vi "SignIn&Out QR Code.vi"(8 "error in (no error)":errorcluster, 11 "Para":T1={"url"="http://data.watersystem.com.cn:50040", "AccessToken"="equip&GbbVkGRBUSaIfhTSjiolTAP8QMM", "mn"="admin", "isSignIn"=FALSE}) -> (0 "error out":errorcluster, 3 "response":T2)   [LabVIEW 2016, in "opSignIn.lvlib"]
uses:
  opSignIn.lvlib
  <vilib>/httpClient/LabVIEWHTTPClient.lvlib
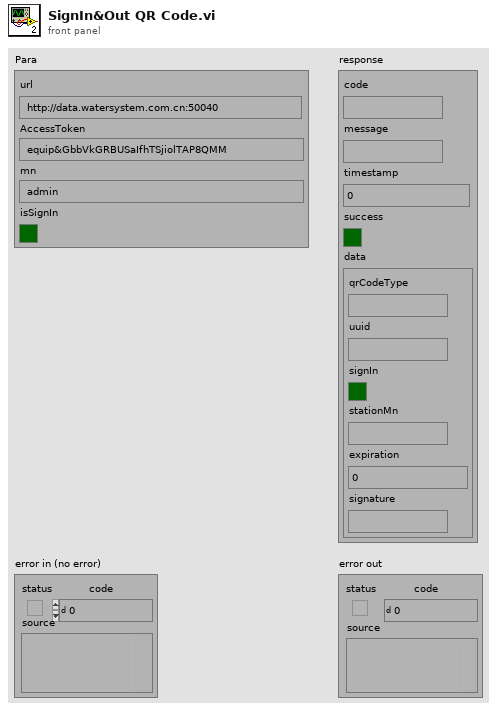
[diagram p1: front panel]
types:
  T1 = cluster{"url":string, "AccessToken":string, "mn":string, "isSignIn":bool}
  T2 = cluster{"code":string, "message":string, "timestamp":u64, "success":bool, "data":cluster{"qrCodeType":string, "uuid":string, "signIn":bool, "stationMn":string, "expiration":u64, "signature":string}}
  T3 = cluster{"code":string, "message":string, "success":bool}
  T4 = typedef "LabVIEWHTTPClient.lvlib/ClientHandle.ctl" = refnum<k1>
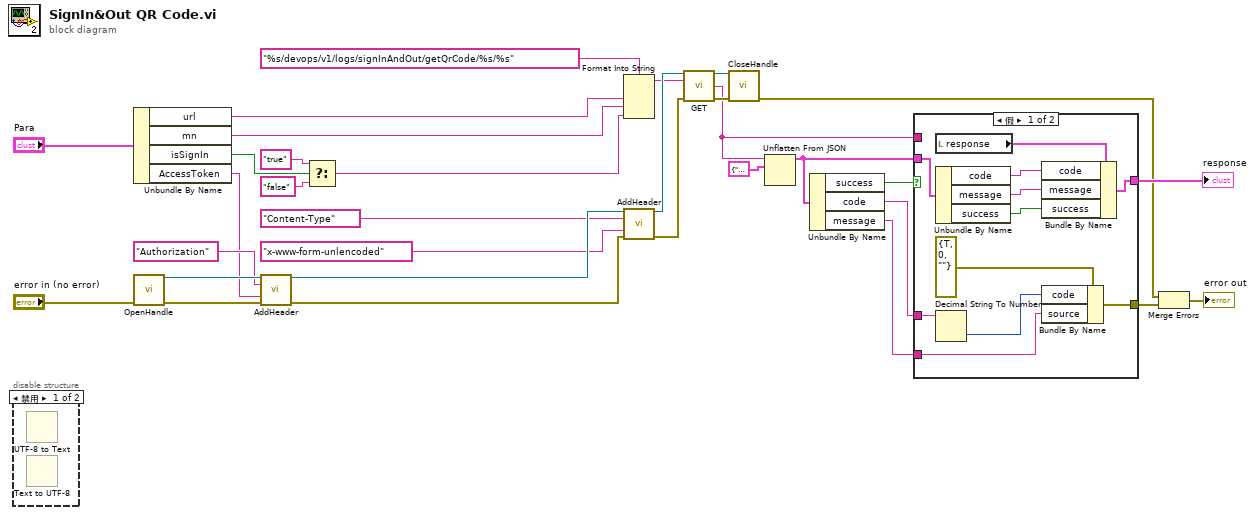
[diagram p0: block diagram]
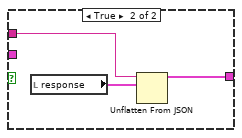
[diagram p2: hidden frame]
diagram:
  n1 = disable-structure shown="禁用" {
    frame Disabled {
      n2 = UTF-8 to Text() -> ()  [unwired: 3 in, 2 out]
      n3 = Text to UTF-8() -> ()  [unwired: 3 in, 2 out]
    }
    frame Enabled {
    }
  }
  n4 = Unbundle By Name("Para") -> ("url"=w1:string, "mn"=w14:string, "isSignIn"=w13:bool, "AccessToken"=w12:string)
  n5 = call <vilib>:"OpenHandle.vi"("error in (no error)"="error in (no error)") -> ("client handle out"=w32:T4, "error out"=w31:errorcluster)  [unwired: 13 in]
  n6 = call <vilib>:"AddHeader.vi"("client handle"=w32, "header"="Authorization", "value"=w12, "error in (no error)"=w31) -> ("client handle out"=w28:T4, "error out"=w27:errorcluster)  [unwired: 10 in]
  n7 = Select(t="true", s=w13, f="false") -> (s? t:f=w16:string)
  n8 = Format Into String(format string="%s/devops/v1/logs/signInAndOut/getQrCode/%s/%s" ("url"), w1, w14, w16) -> (resulting string=w19:string)  [unwired: 2 in, 1 out]
  n9 = call <vilib>:"AddHeader.vi"("client handle"=w28, "header"="Content-Type", "value"="x-www-form-unlencoded", "error in (no error)"=w27) -> ("client handle out"=w24:T4, "error out"=w23:errorcluster)  [unwired: 10 in]
  n10 = call <vilib>:"GET.vi"("client handle"=w24, "url"=w19, "error in (no error)"=w23) -> ("client handle out"=w22:T4, "body"=w8:string, "error out"=w21:errorcluster)  [unwired: 9 in, 1 out]
  n11 = call <vilib>:"CloseHandle.vi"("client handle"=w22, "error in (no error)"=w21) -> ("error out"=w4:errorcluster)  [unwired: 13 in]
  n12 = Unflatten From JSON(JSON string=w8, type and defaults=T3 {"code"="", "message"="", "success"=FALSE} ("response 2")) -> (value=w7:T3)  [unwired: 5 in, 1 out]
  n13 = Unbundle By Name(w7) -> ("success"=w10:bool, "code"=w6:string, "message"=w5:string)
  n14 = case shown="假" w10 {
    tunnel: [w42 w45] -> w9
    tunnel: w8 -> [_ w44]
    tunnel: w7 -> [w41 _]
    tunnel: w6 -> [w35 _]
    tunnel: w5 -> [w36 _]
    tunnel: [w33 _] -> w3
    frame False {
      n15 = local read "response"() -> (w43:T2)
      n16 = Unbundle By Name(w41) -> ("code"=w40:string, "message"=w39:string, "success"=w38:bool)
      n17 = Decimal String To Number(string=w35) -> (number=w34:i32)  [unwired: 2 in, 1 out]
      n18 = Bundle By Name(cluster=w43, "code"=w40, "message"=w39, "success"=w38) -> (w42:T2)
      n19 = Bundle By Name(cluster=errorcluster {"status"=TRUE, "code"=0, "source"=""} ("错误常量"), "code"=w34, "source"=w36) -> (w33:errorcluster)
    }
    frame True {
      n20 = local read "response"() -> (w46:T2)
      n21 = Unflatten From JSON(JSON string=w44, type and defaults=w46) -> (value=w45:T2)  [unwired: 5 in, 1 out]
    }
  }
  "response" <- w9
  n22 = Merge Errors(w4, w3) -> (→"error out":errorcluster)
